vi "Abort Single Point Source-Single.vi"(8 "error in":errorcluster, 11 "Abort Single Point - Single":T1) -> (0 "error out":errorcluster)   [LabVIEW 2021]
doc: "Abort the single point. In case of error resets the device."
uses:
  controls/Abort Single Point-Single.ctl
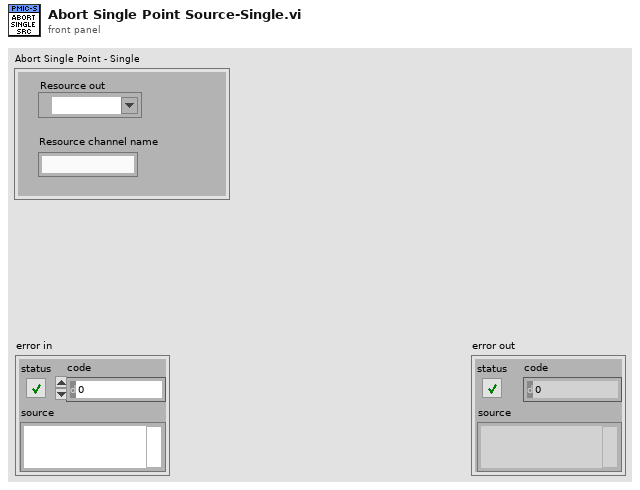
[diagram p1: front panel]
types:
  T1 = typedef "Abort Single Point-Single.ctl" = cluster{"Resource out":refnum<k15>, "Resource channel name":string}
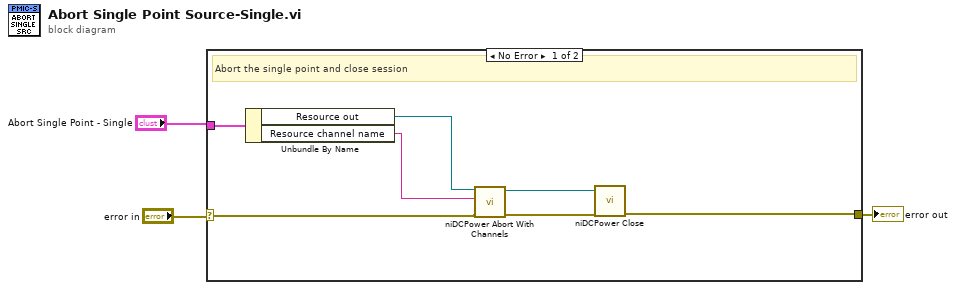
[diagram p0: block diagram]
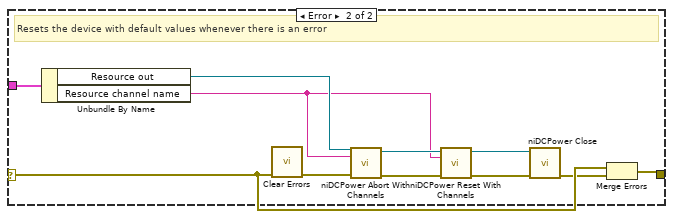
[diagram p2: hidden frame]
diagram:
  n1 = case shown="No Error" "error in" {
    selector: "error in" -> [w4 w13]
    tunnel: "Abort Single Point - Single" -> [w10 w21]
    tunnel: [w5 w11] -> w1
    frame No Error {
      # "Abort the single point and close session"
      n2 = Unbundle By Name(w10) -> ("Resource out"=w7:refnum<k15>, "Resource channel name"=w6:string)
      n3 = call <instrlib>:"niDCPower Abort With Channels.vi"("error in (no error)"=w4, "channel name"=w6, "instrument handle"=w7) -> ("error out"=w9:errorcluster, "instrument handle out"=w8:refnum<k15>)  [unwired: 7 in]
      n4 = call <instrlib>:"niDCPower Close.vi"("error in (no error)"=w9, "instrument handle"=w8) -> ("error out"=w5:errorcluster)  [unwired: 9 in]
    }
    frame Error {
      # "Resets the device with default values whenever there is an error"
      n5 = Unbundle By Name(w21) -> ("Resource out"=w16:refnum<k15>, "Resource channel name"=w15:string)
      n6 = call <vilib>:"Clear Errors.vi"("error in (no error)"=w13) -> ("error out"=w14:errorcluster)  [unwired: 5 in, 1 out]
      n7 = call <instrlib>:"niDCPower Abort With Channels.vi"("error in (no error)"=w14, "channel name"=w15, "instrument handle"=w16) -> ("error out"=w20:errorcluster, "instrument handle out"=w19:refnum<k15>)  [unwired: 7 in]
      n8 = call <instrlib>:"niDCPower Reset With Channels.vi"("error in (no error)"=w20, "channel name"=w15, "instrument handle"=w19) -> ("error out"=w18:errorcluster, "instrument handle out"=w17:refnum<k15>)  [unwired: 7 in]
      n9 = call <instrlib>:"niDCPower Close.vi"("error in (no error)"=w18, "instrument handle"=w17) -> ("error out"=w12:errorcluster)  [unwired: 9 in]
      n10 = Merge Errors(w13, w12) -> (w11:errorcluster)
    }
  }
  "error out" <- w1
